vi "Clamp.vi"(8 "error in (no error)":errorcluster, 11 "Instrument.1820 in":refnum<class "Instrument.Oxford1820.lvclass">) -> (0 "error out":errorcluster, 2 "Response":string, 3 "Instrument.1820 in":refnum<class "Instrument.Oxford1820.lvclass">)   [LabVIEW 2019, in "Instrument.Oxford1820.lvclass"]
uses:
  Instrument.Oxford1820.lvclass
  Typedefs/Instrument.Oxford1820.protectedCommands-enum.ctl
  0ae21551-d9ab-4416-a173-b42d0019b003.vi/b25308ce-79e2-417a-a5cf-67f84cfbe3d3.vi
  0ae21551-d9ab-4416-a173-b42d0019b003.vi/2f4dfc3a-5cd2-4273-83dc-46227e2f899b.vi
  <vilib>/Utility/Data Type/Get Type Information.vi
  <vilib>/JDP Science/JSONtext/JSON text to Variant.vi
  <vilib>/JDP Science/JSONtext/LVClass Serializer/JSONtext LVClass Serializer.lvclass
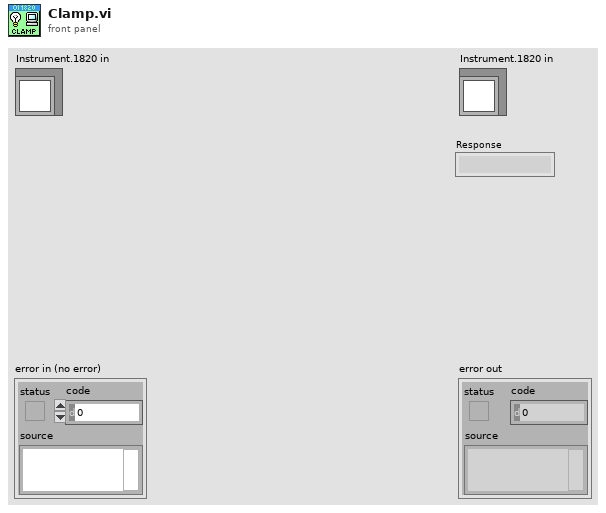
[diagram p1: front panel]
types:
  T1 = typedef "Instrument.Oxford1820.lvclass/Instrument.Oxford1820.protectedCommands-enum.ctl" = enum16{"Hold", "RampToSet", "RampToZero", "Clamp", "setTarget", "setSwitchHeat", "setLambda", "setFillMode", "setNeedleValve", "getStatus", "getTarget", "getSwitchHeat", "getPSUField", "setSequenceStatus"}
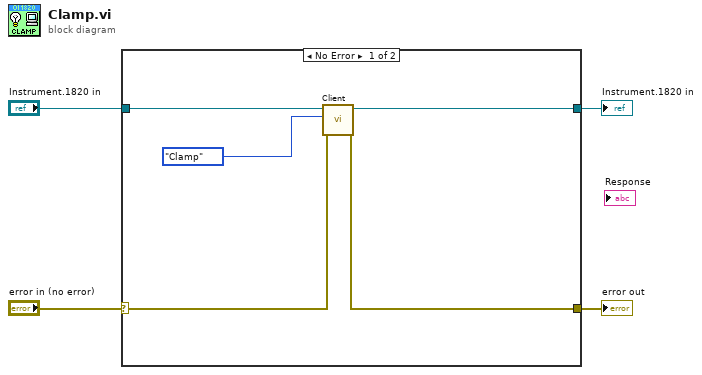
[diagram p0: block diagram]
diagram:
  n1 = case shown="No Error" "error in (no error)" {
    selector: "error in (no error)" -> [w7 w11]
    tunnel: [w5 w11] -> w3
    tunnel: [w6 w10] -> w1
    tunnel: "Instrument.1820 in" -> [w8 w10]
    frame No Error {
      n2 = call-dynamic "Client.vi"("error in (no error)"=w7, "Command in"=Instrument.Oxford1820.protectedCommands-enum."Clamp" ("protectedCommands"), "Instrument in"=w8) -> ("error out"=w5:errorcluster, "Instrument out"=w6:refnum<class "Instrument.Oxford1820.lvclass">)  [unwired: 5 in, 2 out]
    }
    frame Error {
    }
  }
  "error out" <- w3
  "Instrument.1820 in" <- w1
